vi "Update Beam Separations.vi"() -> ()   [LabVIEW 2022 SP3]
uses:
  File/Setup_Filetype.ctl
panel:
  out "Filename Out":path
  out "error out":errorcluster
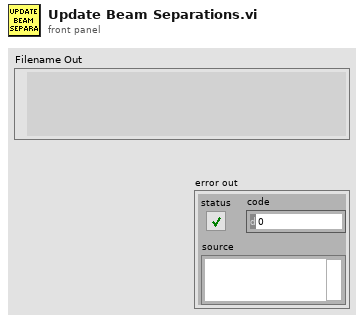
[diagram p1: front panel]
types:
  T1 = typedef "Setup_Filetype.ctl" = enum16{"Measurement Setups", "Calibration Setups", "General", "Results File Plotter Setups", "Speed Calib Tweaks"}
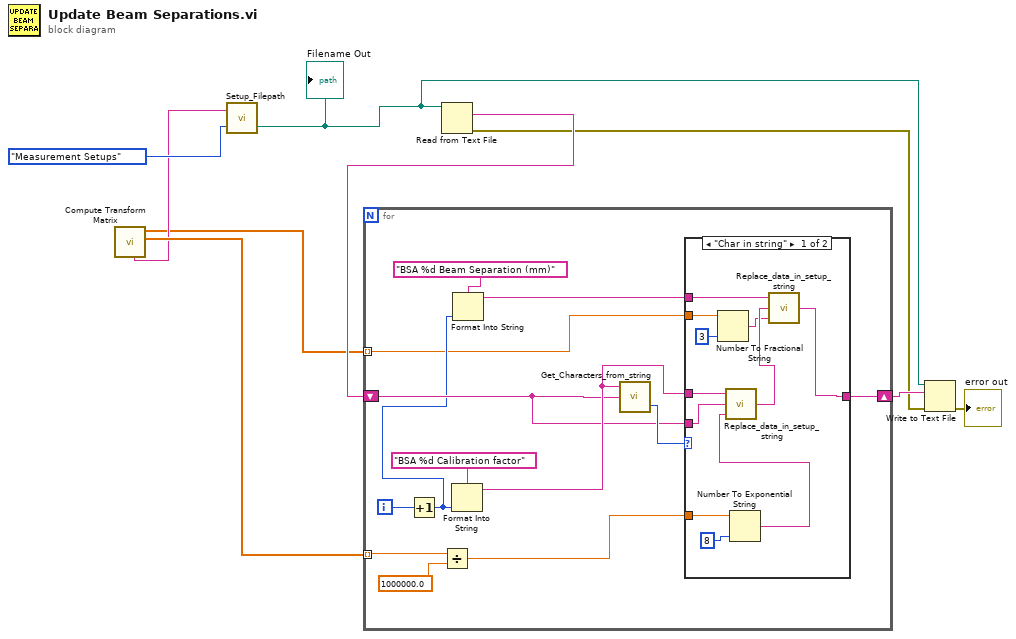
[diagram p0: block diagram]
diagram:
  n1 = call "Compute Transform Matrix.vi"() -> ("Calibration Factor m/s per MHz"=w4:dbl[], "Beam Separations"=w1:dbl[], "Meas Setup File"=w3:string)  [unwired: 6 in, 3 out]
  n2 = call "Setup_Filepath.vi"("Setup File Type"=Setup_Filetype."Measurement Setups", "Filename in"=w3) -> ("Filename Out"=w2:path)  [unwired: 1 out]
  "Filename Out" <- w2
  n3 = Read from Text File(file (use dialog)=w2) -> (text=w8:string, error out=w6:errorcluster)  [unwired: 3 in, 2 out]
  n4 = for {
    shift-right: [w18] -> w7
    shift-left: w8 -> [w17]
    tunnel: w4 -> [w16] mode=indexing
    tunnel: w1 -> [w11] mode=indexing
    i -> [w21]
    n5 = Increment(x=w21) -> (x+1=w12:i32)
    n6 = Divide(x=w16, y=1000000.0) -> (x/y=w14:dbl)
    n7 = Format Into String(format string="BSA %d Calibration factor", w12) -> (resulting string=w20:string)  [unwired: 2 in, 1 out]
    n8 = Format Into String(format string="BSA %d Beam Separation (mm)", w12) -> (resulting string=w10:string)  [unwired: 2 in, 1 out]
    n9 = call "Get_Characters_from_string.vi"("Input string"=w17, "Variable name"=w20) -> ("Status"=w19:enum16{"Char in string", "Char not in string"})  [unwired: 1 in, 1 out]
    n10 = case shown="\"Char in string\"" w19 {
      tunnel: w20 -> [w33 _]
      tunnel: [w27 w34] -> w18
      tunnel: w17 -> [w32 w34]
      tunnel: w14 -> [w30 _]
      tunnel: w11 -> [w25 _]
      tunnel: w10 -> [w23 _]
      frame "Char in string" {
        n11 = Number To Fractional String(number=w25, precision (6)=i16 3) -> (F-format string=w24:string)  [unwired: 2 in]
        n12 = Number To Exponential String(number=w30, precision (6)=i16 8) -> (E-format string=w29:string)  [unwired: 2 out]
        n13 = call "Replace_data_in_setup_string.vi"("New data string"=w29, "Input string"=w32, "Variable name"=w33) -> ("Appended string"=w28:string)
        n14 = call "Replace_data_in_setup_string.vi"("New data string"=w24, "Input string"=w28, "Variable name"=w23) -> ("Appended string"=w27:string)
      }
      frame "Char not in string" {
      }
    }
  }
  n15 = Write to Text File(file (use dialog)=w2, text=w7, error in=w6) -> (error out=→"error out":errorcluster)  [unwired: 1 in, 2 out]
